vi "GetDateAndTime.vi"() -> (0 "Day_clean":string, 1 "Year_clean":string, 2 "Month_clean":string, 3 "Date":string, 4 "time":string)   [LabVIEW 2018]
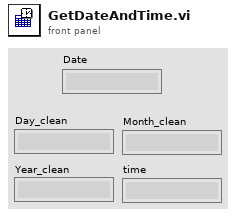
[diagram p1: front panel]
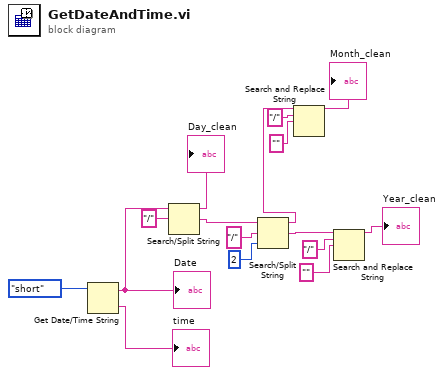
[diagram p0: block diagram]
diagram:
  n1 = Get Date/Time String(date format (0)=enum16{"short", "long", "abbreviated"}."short") -> (date string=w15:string, time string=→"time":string)  [unwired: 2 in]
  "Date" <- w15
  n2 = Search/Split String(string=w15, search string/char (-)="/") -> (substring before match=→"Day_clean":string, match + rest of string=w13:string)  [unwired: 1 in, 1 out]
  n3 = Search/Split String(string=w13, search string/char (-)="/", offset (0)=2) -> (substring before match=w4:string, match + rest of string=w1:string)  [unwired: 1 out]
  n4 = Search and Replace String(input string=w4, search string="/", replace string="" ("replace string (\"\")")) -> (result string=→"Month_clean":string)  [unwired: 5 in, 3 out]
  n5 = Search and Replace String(input string=w1, search string="/", replace string="" ("replace string (\"\")")) -> (result string=→"Year_clean":string)  [unwired: 5 in, 3 out]
